vi "Date Format Check.vi"(8 "error in (no error)":errorcluster, 11 "Formated Date":string) -> (0 "error out":errorcluster, 3 "Formated?":bool)   [LabVIEW 2016, in "User Interface.lvlib"]
uses:
  User Interface.lvlib
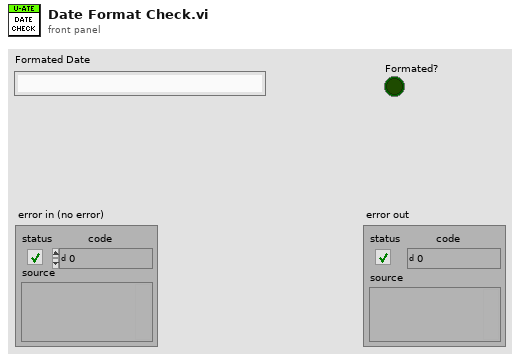
[diagram p1: front panel]
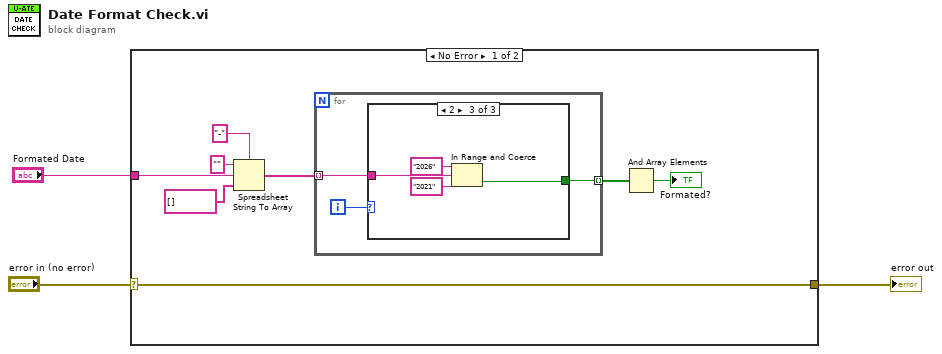
[diagram p0: block diagram]
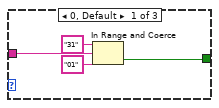
[diagram p2: hidden frame]
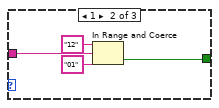
[diagram p3: hidden frame]
diagram:
  n1 = case shown="No Error" "error in (no error)" {
    selector: "error in (no error)" -> [w6 w27]
    tunnel: [w6 w27] -> w2
    tunnel: "Formated Date" -> [w8 _]
    frame No Error {
      n2 = Spreadsheet String To Array(delimiter (Tab)="-", format string="", spreadsheet string=w8, array type (2D Dbl)=string[] []) -> (array=w7:string[])
      n3 = for {
        tunnel: w7 -> [w13] mode=indexing
        tunnel: [w12] -> w5 mode=indexing
        i -> [w14]
        n4 = case shown="2" w14 {
          tunnel: w13 -> [w18 w22 w26]
          tunnel: [w15 w19 w23] -> w12
          frame 0, Default {
            n5 = In Range and Coerce(upper limit="31", x=w18, lower limit="01") -> (In Range?=w15:bool)  [unwired: 1 out]
          }
          frame 1 {
            n6 = In Range and Coerce(upper limit="12", x=w22, lower limit="01") -> (In Range?=w19:bool)  [unwired: 1 out]
          }
          frame 2 {
            n7 = In Range and Coerce(upper limit="2026", x=w26, lower limit="2021") -> (In Range?=w23:bool)  [unwired: 1 out]
          }
        }
      }
      n8 = And Array Elements(Boolean array=w5) -> (logical AND=→"Formated?":bool)
    }
    frame Error {
    }
  }
  "error out" <- w2
